vi "Register for SHV Events.vi"(7 "Control Refs":T2, 8 "error in (no error)":errorcluster, 10 "Register for":T1) -> (0 "error out":errorcluster, 3 "Containers SHV change notification":refnum<user-event>)   [LabVIEW 2015]
uses:
  Controls/FP Control Refs Cluster.ctl
  Controls/Liquid N Valve Ref Cluster.ctl
  Controls/Main Line Valve Ref Cluster.ctl
  Controls/Sample Valve Refs.ctl
  Controls/Syringe Ctrl Refs.ctl
  Controls/Register For Notifications Enumerator.ctl
  <vilib>/lvdsc/NI_DSC.lvlib
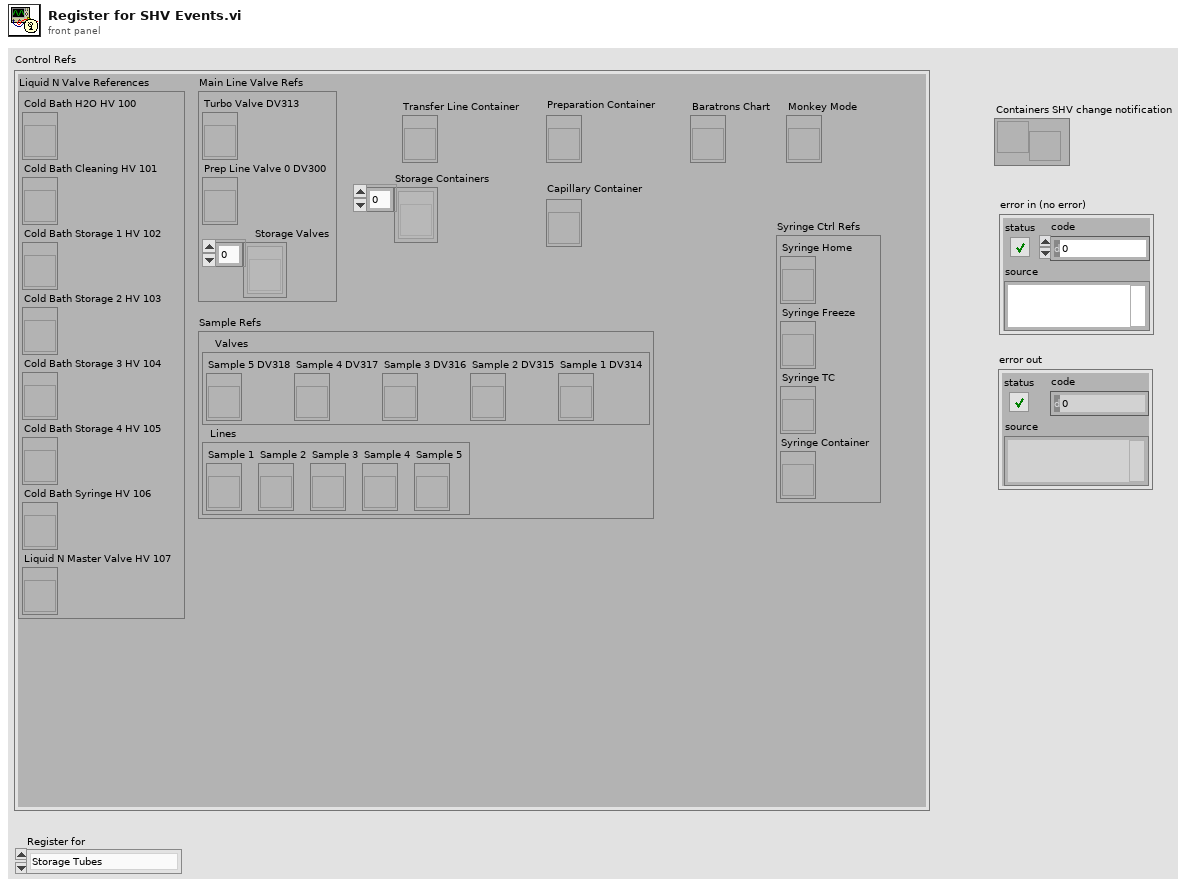
[diagram p1: front panel]
types:
  T1 = typedef "Register For Notifications Enumerator.ctl" = enum16{"Storage Tubes", "Storage Valves", "Sample Lines", "Syringe Container", "Capillary Container", "Preparation Line"}
  T2 = typedef "FP Control Refs Cluster.ctl" = cluster{"Liquid N Valve References":T3, "Main Line Valve Refs":T4, "Transfer Line Container":refnum<vi>, "Storage Containers":refnum<vi>[], "Sample Refs":T5, "Syringe Ctrl Refs ":T6, "Baratrons Chart":refnum<vi>, "Capillary Container":refnum<vi>, "Preparation Container":refnum<vi>, "Monkey Mode":refnum<vi>}
  T3 = typedef "Liquid N Valve Ref Cluster.ctl" = cluster{"Cold Bath H2O HV 100":refnum<vi>, "Cold Bath Cleaning HV 101":refnum<vi>, "Cold Bath Storage 1 HV 102":refnum<vi>, "Cold Bath Storage 2 HV 103":refnum<vi>, "Cold Bath Storage 3 HV 104":refnum<vi>, "Cold Bath Storage 4 HV 105":refnum<vi>, "Cold Bath Syringe HV 106":refnum<vi>, "Liquid N Master Valve HV 107":refnum<vi>}
  T4 = typedef "Main Line Valve Ref Cluster.ctl" = cluster{"Turbo Valve DV313":refnum<vi>, "Prep Line Valve 0 DV300":refnum<vi>, "Storage Valves":refnum<vi>[]}
  T5 = typedef "Sample Valve Refs.ctl" = cluster{"Valves":cluster{"Sample 5 DV318":refnum<vi>, "Sample 4 DV317":refnum<vi>, "Sample 3 DV316":refnum<vi>, "Sample 2 DV315":refnum<vi>, "Sample 1 DV314":refnum<vi>}, "Lines":cluster{"Sample 1":refnum<vi>, "Sample 2":refnum<vi>, "Sample 3":refnum<vi>, "Sample 4":refnum<vi>, "Sample 5":refnum<vi>}}
  T6 = typedef "Syringe Ctrl Refs.ctl" = cluster{"Syringe Home":refnum<vi>, "Syringe Freeze":refnum<vi>, "Syringe TC":refnum<vi>, "Syringe Container":refnum<vi>}
  T7 = cluster{"Sample 1":refnum<vi>, "Sample 2":refnum<vi>, "Sample 3":refnum<vi>, "Sample 4":refnum<vi>, "Sample 5":refnum<vi>}
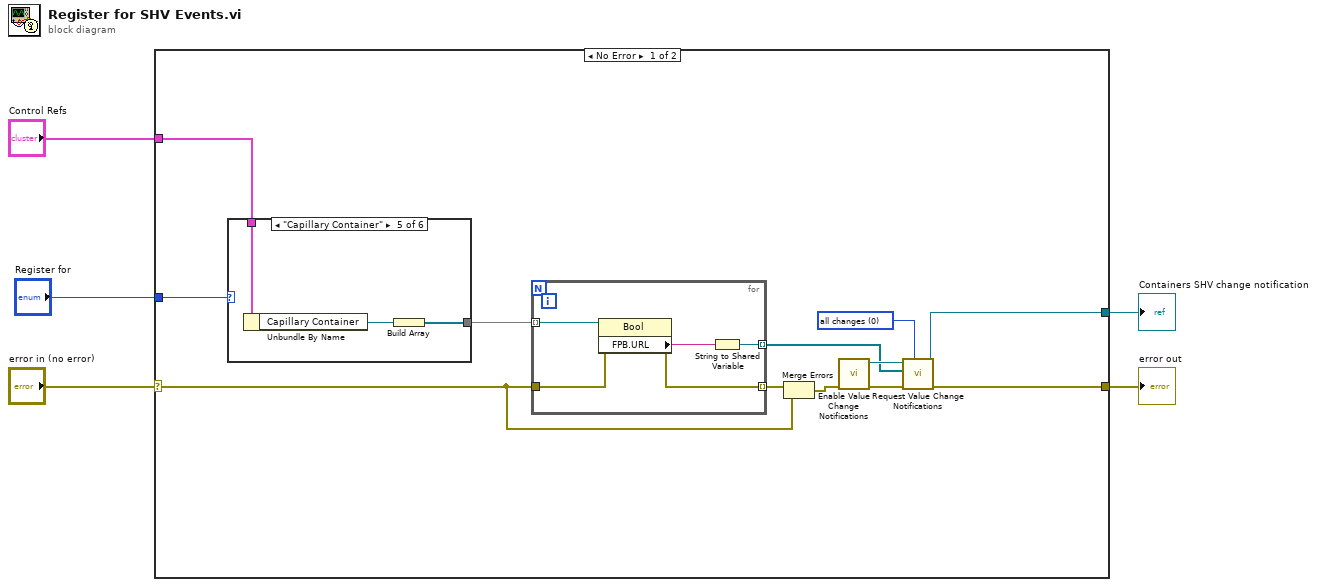
[diagram p0: block diagram]
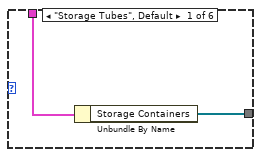
[diagram p2: hidden frame]
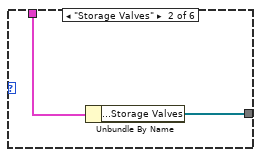
[diagram p3: hidden frame]
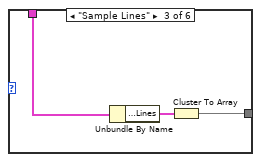
[diagram p4: hidden frame]
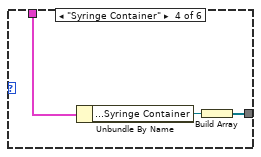
[diagram p5: hidden frame]
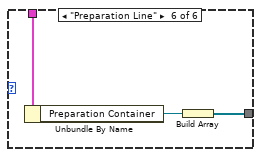
[diagram p6: hidden frame]
diagram:
  n1 = case shown="No Error" "error in (no error)" {
    selector: "error in (no error)" -> [w8 w39]
    tunnel: [w7 w39] -> w4
    tunnel: "Control Refs" -> [w9 _]
    tunnel: [w10 _] -> w2
    tunnel: "Register for" -> [w6 _]
    frame No Error {
      w11 = u16 0 items=["all changes", "value changes only"] ("request changes (all changes)")
      n2 = case shown="\"Capillary Container\"" w6 {
        tunnel: [w19 w21 w22 w25 w28 w31] -> w17
        tunnel: w9 -> [w18 w20 w23 w27 w30 w33]
        frame "Storage Tubes", Default {
          n3 = Unbundle By Name(w18) -> ("Storage Containers"=w19:refnum<vi>[])
        }
        frame "Storage Valves" {
          n4 = Unbundle By Name(w20) -> ("Main Line Valve Refs.Storage Valves"=w21:refnum<vi>[])
        }
        frame "Sample Lines" {
          n5 = Unbundle By Name(w23) -> ("Sample Refs.Lines"=w24:T7)
          n6 = Cluster To Array(cluster=w24) -> (array=w22:refnum<vi>[])
        }
        frame "Syringe Container" {
          n7 = Unbundle By Name(w27) -> ("Syringe Ctrl Refs.Syringe Container"=w26:refnum<vi>)
          n8 = Build Array(w26) -> (w25:refnum<vi>[])
        }
        frame "Capillary Container" {
          n9 = Unbundle By Name(w30) -> ("Capillary Container"=w29:refnum<vi>)
          n10 = Build Array(w29) -> (w28:refnum<vi>[])
        }
        frame "Preparation Line" {
          n11 = Unbundle By Name(w33) -> ("Preparation Container"=w32:refnum<vi>)
          n12 = Build Array(w32) -> (w31:refnum<vi>[])
        }
      }
      n13 = for {
        tunnel: w8 -> [w37]
        tunnel: w17 -> [w38] mode=indexing
        tunnel: [w35] -> w16 mode=indexing
        tunnel: [w34] -> w12 mode=indexing
        n14 = property class="Bool"(reference=w38, error in=w37) -> (error out=w35:errorcluster, "FPB.URL"=w36:string)  [unwired: 1 out]
        n15 = String to Shared Variable(0:w36) -> (2:w34:refnum<k21>)  [unwired: 1 out]
      }
      n16 = Merge Errors(w16, w8) -> (w15:errorcluster)
      n17 = call <vilib>:"Enable Value Change Notifications.vi"("error in (no error)"=w15) -> ("error out"=w14:errorcluster, "shared variable value change notification"=w13:refnum<user-event>)  [unwired: 9 in]
      n18 = call <vilib>:"Request Value Change Notifications.vi"("request changes (all changes)"=w11, "error in (no error)"=w14, "shared variables"=w12, "notification refnum"=w13) -> ("error out"=w7:errorcluster, "shared variable value change notification"=w10:refnum<user-event>)  [unwired: 5 in, 1 out]
    }
    frame Error {
    }
  }
  "error out" <- w4
  "Containers SHV change notification" <- w2
